vi "Image Dual Threshold [SGL].vi"(8 "error in (no error)":errorcluster, 9 "Range":cluster{"Lower value":sgl, "Upper value":sgl}={"Lower value"=128.0, "Upper value"=255.0} {"Upper value" format="%.2f"; "Lower value" format="%.2f"}, 10 "Image Dst":T2, 11 "Image Src":T2) -> (0 "error out":errorcluster, 1 "CPU (s)":dbl, 3 "Image Dst Out":T2)   [LabVIEW 2021, in "Image.lvlib"]
doc: "Sets the out-of-range values of <B>Image Src</B>s to range min or max.s\n\nIf <B>Image Dst</B> is not provided, <B>Image Src</B> is used as the destination."
uses:
  Image.lvlib
  <vilib>/vision/Image Controls.llb/IMAQ Image.ctl
  <vilib>/vision/EDVR.llb/IMAQ ImageToEDVR 2D SGL.vi
  Time/Time.lvlib
panel:
  out "Line Info":T1
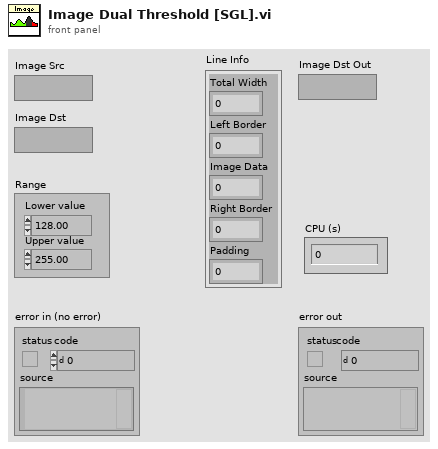
[diagram p1: front panel]
types:
  T1 = cluster{"Total Width":u32, "Left Border":u32, "Image Data":u32, "Right Border":u32, "Padding":u32}
  T2 = typedef "IMAQ Image.ctl" = refnum<image>
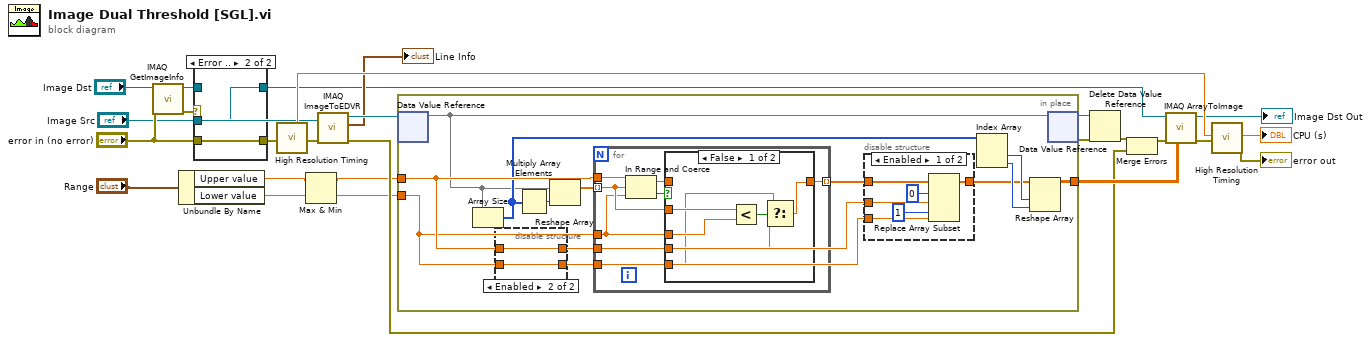
[diagram p0: block diagram]
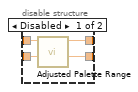
[diagram p2: hidden frame]
diagram:
  n1 = call "IMAQ GetImageInfo"("error in (no error)"="error in (no error)", "Image"="Image Dst") -> ("error out"=w10:errorcluster)  [unwired: 2 in, 7 out]
  n2 = Unbundle By Name("Range") -> ("Upper value"=w4:sgl, "Lower value"=w3:sgl)
  n3 = case shown="Error .." w10 {
    selector: w10 -> [w26 _]
    tunnel: "Image Dst" -> [w27 _]
    tunnel: [w27 w28] -> w8
    tunnel: "error in (no error)" -> [_ w29]
    tunnel: [w26 w29] -> w6
    tunnel: "Image Src" -> [_ w28]
    frame No Error {
    }
    frame Error {
    }
  }
  n4 = call "High Resolution Timing.vi"("Error In"=w6) -> ("elapsed (relative) seconds"=w19:dbl, "Error Out"=w22:errorcluster)  [unwired: 16 in, 1 out]
  n5 = Max & Min(x=w4, y=w3) -> (max(x,y)=w2:sgl, min(x,y)=w1:sgl)
  n6 = call-poly <vilib>:"IMAQ ImageToEDVR.vi"("error in (no error)"=w22, "Image"="Image Src") -> ("error out"=w15:errorcluster, "Line Info"=→"Line Info":T1, "EDVR 2D SGL"=w25:refnum<data-value>)  [unwired: 7 in]
  n7 = in-place {
    in-place-border: w2 -> [w41]
    in-place-border: w1 -> [w40]
    in-place-border: [w42] -> w21
    n8 = in-place-dvr #1(w25) -> (w30:sgl[][])  [unwired: 1 out]
    n9 = Array Size(array=w30) -> (size(s)=w38:i32[])
    n10 = disable-structure shown="Enabled" {
      disable-tunnel: w41 -> [w46 w48]
      disable-tunnel: w40 -> [w45 w47]
      disable-tunnel: [w44 w48] -> w32
      disable-tunnel: [w43 w47] -> w31
      frame Disabled {
        n11 = call "Adjusted Palette Range.vi"("Image Min"=w45, "Image Max"=w46) -> ("Palette Range Min"=w43:sgl, "Palette Range Max"=w44:sgl)  [unwired: 7 in, 1 out]
      }
      frame Enabled {
      }
    }
    n12 = Multiply Array Elements(1:w38) -> (0:w33:i32)
    n13 = Reshape Array(w30, w33) -> (w39:sgl[])
    n14 = for {
      tunnel: w39 -> [w59] mode=indexing
      tunnel: w41 -> [w63]
      tunnel: w40 -> [w58]
      tunnel: [w60] -> w35 mode=indexing
      tunnel: w32 -> [w57]
      tunnel: w31 -> [w56]
      n15 = In Range and Coerce(upper limit=w63, x=w59, lower limit=w58) -> (coerced(x)=w61:sgl, In Range?=w62:bool)
      n16 = case shown="False" w62 {
        tunnel: w61 -> [_ w70]
        tunnel: [w66 w70] -> w60
        tunnel: w59 -> [w69 _]
        tunnel: w58 -> [w68 _]
        tunnel: w57 -> [w65 _]
        tunnel: w56 -> [w64 _]
        frame False {
          n17 = Less?(x=w69, y=w68) -> (x < y?=w67:bool)
          n18 = Select(t=w64, s=w67, f=w65) -> (s? t:f=w66:sgl)
        }
        frame True {
        }
      }
    }
    n19 = disable-structure shown="Enabled" {
      disable-tunnel: w35 -> [w54 w55]
      disable-tunnel: [w53 w55] -> w34
      disable-tunnel: w32 -> [w49 _]
      disable-tunnel: w31 -> [w50 _]
      frame Enabled {
        n20 = Replace Array Subset(array=w54, new element #1=w49, index #1=0 ("index"), new element #2=w50, index #2=1 ("index")) -> (w53:sgl[])
      }
      frame Disabled {
      }
    }
    n21 = Index Array(array=w38) -> (element #1=w37:i32, element #2=w36:i32)  [unwired: 2 in]
    n22 = Reshape Array(w34, w37, w36) -> (w42:sgl[][])
    n23 = in-place-dvr #1(w30) -> (w23:refnum<data-value>, w11:errorcluster)
  }
  n24 = Delete Data Value Reference(data value reference=w23, error in=w11) -> (error out=w16:errorcluster)  [unwired: 1 out]
  n25 = Merge Errors(w16, w15) -> (w17:errorcluster)
  n26 = call "IMAQ ArrayToImage"("Image Pixels (Float)"=w21, "error in (no error)"=w17, "Image"=w8) -> ("error out"=w14:errorcluster, "Image Out"=→"Image Dst Out":T2)  [unwired: 7 in]
  n27 = call "High Resolution Timing.vi"("relative seconds (NaN)"=w19, "Error In"=w14) -> ("elapsed (relative) seconds"=→"CPU (s)":dbl, "Error Out"=→"error out":errorcluster)  [unwired: 15 in, 1 out]
